vi "Sort 2D Array.vi"(1 "initialized array":string[][](array[string])) -> (0 "Array":string[][](array[string]))   [LabVIEW 2012]
doc: "This vi sorts a two-column array in reference to its first column."
panel:
  # "Purpose: This vi sorts a two-column array in reference to its first column."
  # "Instructions: Input a 2D array and then execute the program."
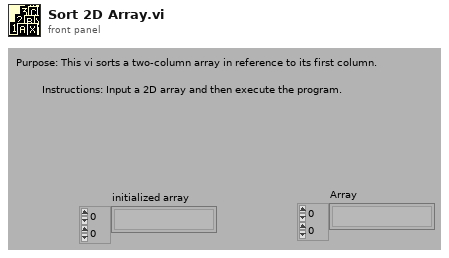
[diagram p1: front panel]
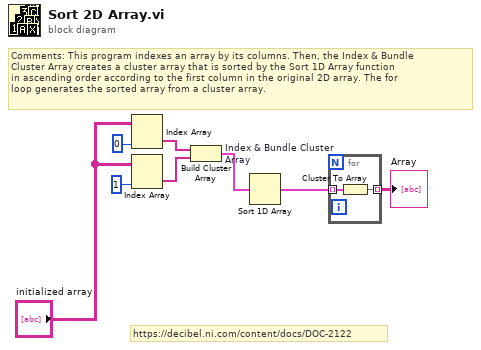
[diagram p0: block diagram]
diagram:
  # "https://decibel.ni.com/content/docs/DOC-2122"
  # "Comments: This program indexes an array by its columns. Then, the Index & Bundle\nCluster Array creates a cluster array that is sorted by the Sort 1D Array function\nin ascending order according to the first column in the original 2D array. The for\nloop generates the sorted array from a cluster array."
  n1 = Index Array(array="initialized array", index (col)=0) -> (element=w8:string[])  [unwired: 1 in]
  n2 = Index Array(array="initialized array", index (col)=1) -> (element=w7:string[])  [unwired: 1 in]
  n3 = Build Cluster Array "Index & Bundle Cluster Array"(w8, w7) -> (w6:cluster{string, string}[])
  n4 = Sort 1D Array(array=w6) -> (sorted array=w5:cluster{string, string}[])
  n5 = for {
    tunnel: w5 -> [w10] mode=indexing
    tunnel: [w9] -> w2 mode=indexing
    n6 = Cluster To Array(cluster=w10) -> (array=w9:string[])
  }
  "Array" <- w2
